vi "Equalize_Sub.vi"(8 "error in (no error)":errorcluster, 11 "Image Src":T1) -> (0 "error out":errorcluster, 3 "Image Out":T1(plugin-control))   [LabVIEW 2009]
uses:
  <vilib>/vision/Image Controls.llb/IMAQ Image.ctl
  <vilib>/vision/NI_Vision_Development_Module.lvlib
panel:
  out "Original":T2 {"Standard  Variation" format="%.2f"; "Mean Value" format="%.2f"; "Interval Width" format="%.2f"; "Starting Value" format="%.2f"; "Maximal Value" format="%.2f"; "Minimal Value" format="%.2f"}
  out "Equalized":T2 {"Standard  Variation" format="%.2f"; "Mean Value" format="%.2f"; "Interval Width" format="%.2f"; "Starting Value" format="%.2f"; "Maximal Value" format="%.2f"; "Minimal Value" format="%.2f"}
  out "original":T1(plugin-control)
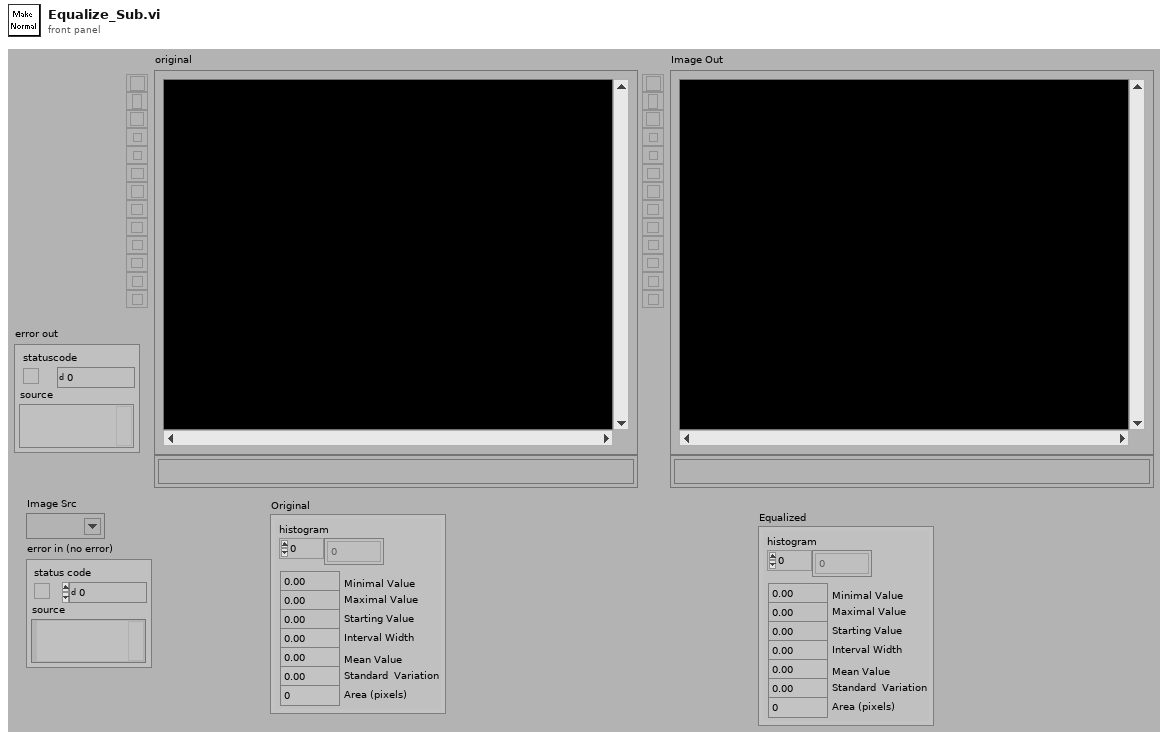
[diagram p1: front panel]
types:
  T1 = typedef "IMAQ Image.ctl" = refnum<image>
  T2 = cluster{"histogram":u32[], "Minimal Value":sgl, "Maximal Value":sgl, "Starting Value":sgl, "Interval Width":sgl, "Mean Value":sgl, "Standard  Variation":sgl, "Area (pixels)":i32}
  T3 = enum32{"Linear", "Log", "Exp", "Square", "Square root", "Power X", "Power 1/X"}
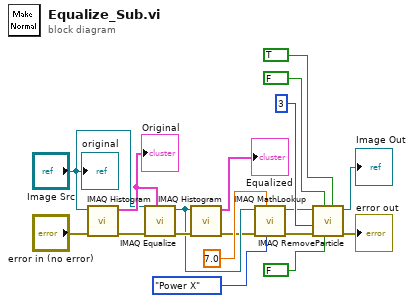
[diagram p0: block diagram]
diagram:
  n1 = call "IMAQ Histogram"("error in (no error)"="error in (no error)", "Image"="Image Src") -> ("error out"=w4:errorcluster, "Histogram Report"=w18:T2)  [unwired: 3 in, 5 out]
  "Original" <- w18
  n2 = call "IMAQ Equalize"("Histogram Report"=w18, "error in (no error)"=w4, "Image Src"="Image Src") -> ("error out"=w17:errorcluster, "Image Dst Out"=w15:T1)  [unwired: 3 in, 4 out]
  n3 = call "IMAQ Histogram"("error in (no error)"=w17, "Image"=w15) -> ("error out"=w3:errorcluster, "Histogram Report"=→"Equalized":T2)  [unwired: 3 in, 5 out]
  n4 = call "IMAQ MathLookup"("Operator"=T3."Power X", "X Value"=sgl 7.0, "error in (no error)"=w3, "Image Src"=w15) -> ("error out"=w8:errorcluster, "Image Dst Out"=w7:T1)  [unwired: 3 in, 3 out]
  n5 = call "IMAQ RemoveParticle"("Connectivity 4/8 (8)"=TRUE, "Low Pass/High Pass (Low)"=FALSE, "Square/Hexa (Square)"=FALSE, "error in (no error)"=w8, "Number of Erosion"=3, "Image Src"=w7) -> ("error out"=→"error out":errorcluster, "Image Dst Out"=→"Image Out":T1)  [unwired: 1 in, 3 out]
  "original" <- "Image Src"
